vi "Simulator SNA Patch Error Code or Caller as Source.vi"(8 "error in (no error)":errorcluster, 9 "string to append to source":string, 10 "operation":u16(ring) items=["patch error code", "patch caller's name"], 11 "error code":i32) -> (0 "error out":errorcluster)   [LabVIEW 2011]
doc: "Call this VI when an error code is first generated (initializing the error out cluster). No need to wire operation input, and the caller's name will be automatically patched as source string.\nAs the error cluster is passed to the next level up, call this VI with only error in/out wired.\n\nThe idea is that the source string gets built up as you pass the error cluster up from the original error source (lowest level subvi) until the highest level (typically those VIs that the user places directly in his diagrams)."
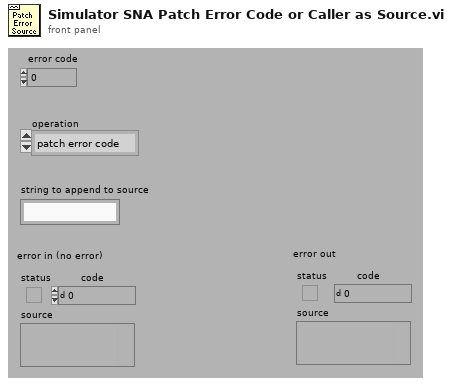
[diagram p1: front panel]
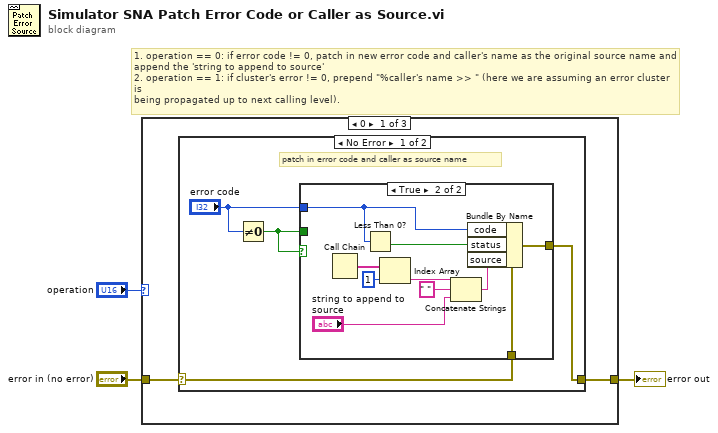
[diagram p0: block diagram]
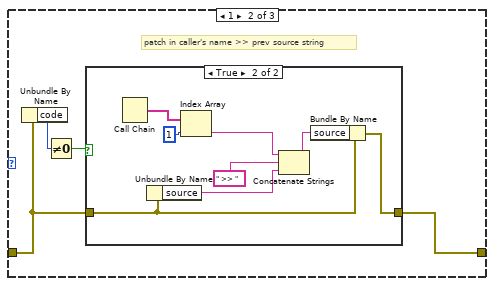
[diagram p4: hidden frame]
diagram:
  # "1. operation == 0: if error code != 0, patch in new error code and caller's name as the original source name and \nappend the 'string to append to source'\n2. operation == 1: if cluster's error != 0, prepend \"%caller's name >> \" (here we are assuming an error cluster is\nbeing propagated up to next calling level)."
  n1 = case shown="0" "operation" {
    tunnel: [w5 w25 w35] -> w2
    tunnel: "error in (no error)" -> [w4 w24 w35]
    frame 0 {
      n2 = case shown="No Error" w4 {
        selector: w4 -> [w6 w21]
        tunnel: [w9 w21] -> w5
        frame No Error {
          # "patch in error code and caller as source name"
          n3 = Not Equal To 0?(x="error code") -> (x != 0?=w7:bool)
          n4 = case shown="True" w7 {
            tunnel: w6 -> [w10 w20]
            tunnel: [w10 w17] -> w9
            tunnel: "error code" -> [_ w16]
            tunnel: w7 -> [_ _]
            frame False {
            }
            frame True {
              n5 = Call Chain() -> (call chain=w19:string[])
              n6 = Less Than 0?(x=w16) -> (x < 0?=w15:bool)
              n7 = Index Array(array=w19, index=1) -> (element=w13:string)
              n8 = Concatenate Strings(w13, " " ("string"), "string to append to source") -> (w11:string)
              n9 = Bundle By Name(cluster=w20, "code"=w16, "status"=w15, "source"=w11) -> (w17:errorcluster)
            }
          }
        }
        frame Error {
          # "input error cluster propagates if we\nare not patching a string to source"
        }
      }
    }
    frame 1 {
      # "patch in caller's name >> prev source string"
      n10 = Unbundle By Name(w24) -> ("code"=w23:i32)
      n11 = Not Equal To 0?(x=w23) -> (x != 0?=w22:bool)
      n12 = case shown="True" w22 {
        tunnel: w24 -> [w26 w33]
        tunnel: [w26 w27] -> w25
        frame False {
        }
        frame True {
          n13 = Call Chain() -> (call chain=w34:string[])
          n14 = Unbundle By Name(w33) -> ("source"=w31:string)
          n15 = Index Array(array=w34, index=1) -> (element=w29:string)
          n16 = Concatenate Strings(w29, " >> ", w31) -> (w28:string)
          n17 = Bundle By Name(cluster=w33, "source"=w28) -> (w27:errorcluster)
        }
      }
    }
    frame Default {
    }
  }
  "error out" <- w2
